vi "Framework-Template.MessageToProcess.vi"(6 "ID":string, 8 "error in (no error)":errorcluster, 9 "Data":variant, 10 "Command":string, 11 "Framework-Template in":refnum<class "Instrument.Framework-Template.lvclass">) -> (0 "error out":errorcluster, 3 "Framework-Template out":refnum<class "Instrument.Framework-Template.lvclass">)   [LabVIEW 2019, in "Instrument.Framework-Template.lvclass"]
doc: "---------------------------------------------------------------\nJKI State Machine Objects™\nhttp://jki.net/state-machine-objects/\nCopyright (C) 2005-2015, JKI <info@jki.net>\nALL RIGHTS RESERVEDJKI State Machine Objects (SMO) 1.0.0.4\nJKI - JKI\nCopyright (c) 2015, JKI"
uses:
  Instrument.Framework-Template.lvclass
  Typedefs/PrivateEvents--Framework-Template.MessageToProcess.ctl
  <userlib>/LevyLab/Instrument Framework/SMOs/RemoteControl/Typedefs/Message--Cluster.ctl
  Instrument.Framework-Template.lvclass/Instrument.Framework-Template.ctl
  <userlib>/LevyLab/Instrument Framework/SMOs/RemoteControl/RemoteControl.lvclass
panel:
  # "For instructions on how to use the JKI State Machine Objects, examples and video tutorials, visit:\nhttp://jki.net/state-machine-objects/\n\nJKI State Machine Objects™\nhttp://jki.net/state-machine-objects/\nCopyright (C) 2005-2015, JKI <info@jki.net>\nALL RIGHTS RESERVED"
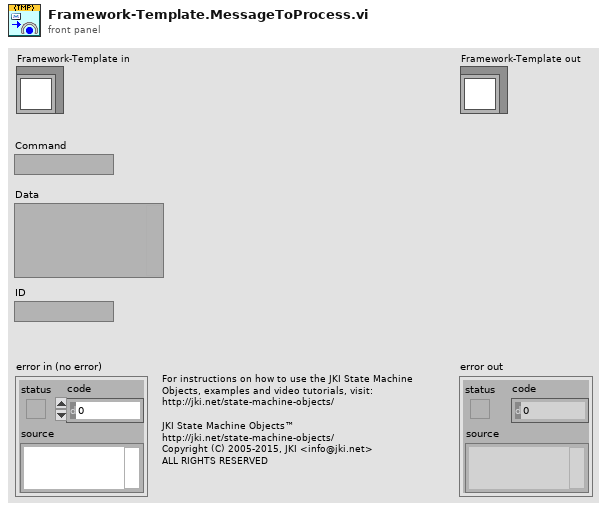
[diagram p1: front panel]
types:
  T1 = typedef "Instrument.Framework-Template.lvclass/PrivateEvents--Framework-Template.MessageToProcess.ctl" = cluster{"Message":T2}
  T2 = typedef "RemoteControl.lvclass/Message--Cluster.ctl" = cluster{"Command":string, "Data":variant, "ID":string}
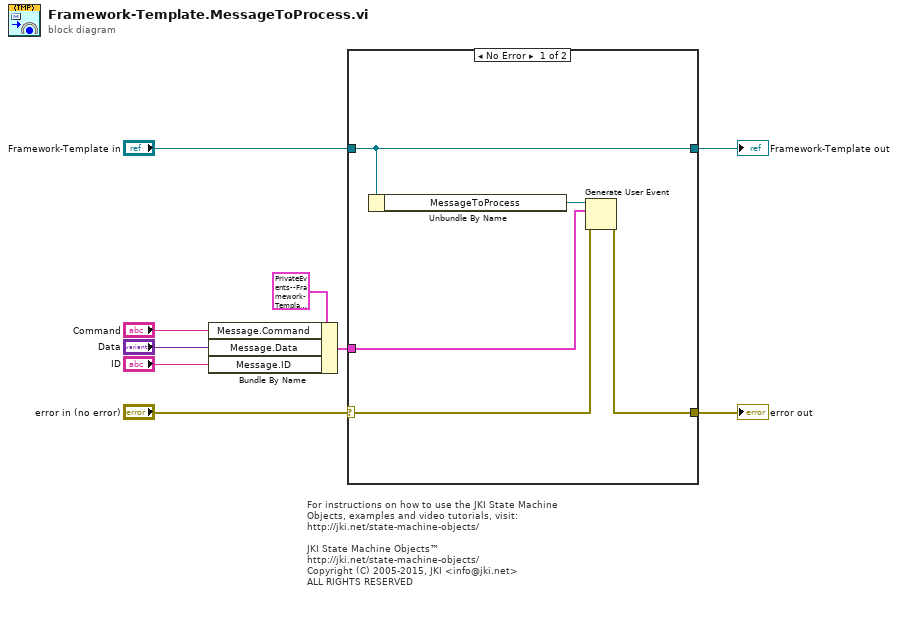
[diagram p0: block diagram]
diagram:
  # "For instructions on how to use the JKI State Machine Objects, examples and video tutorials, visit:\nhttp://jki.net/state-machine-objects/\n\nJKI State Machine Objects™\nhttp://jki.net/state-machine-objects/\nCopyright (C) 2005-2015, JKI <info@jki.net>\nALL RIGHTS RESERVED"
  n1 = Bundle By Name(cluster=T1 {"Message"={"Command"="", "Data"=variant(string ""), "ID"=""}} ("MessageToProcess"), "Message.Command"="Command", "Message.Data"="Data", "Message.ID"="ID") -> (w5:T1)
  n2 = case shown="No Error" "error in (no error)" {
    selector: "error in (no error)" -> [w14 w16]
    tunnel: [w12 w16] -> w8
    tunnel: [w11 w15] -> w9
    tunnel: "Framework-Template in" -> [w11 w15]
    tunnel: w5 -> [w10 _]
    frame No Error {
      n3 = Unbundle By Name(w11) -> ("MessageToProcess"=w13:refnum<user-event>)
      n4 = Generate User Event(user event=w13, event data cluster=w10, error in=w14) -> (error out=w12:errorcluster)  [unwired: 1 in, 1 out]
    }
    frame Error {
    }
  }
  "error out" <- w8
  "Framework-Template out" <- w9
